vi "Start Continuous Acquisition.vi"(6 "lpszRefPath":string, 7 "nMode":u32, 8 "error in (no error)":errorcluster, 9 "pImg":u16[](array[numeric]), 10 "refImg":u16[](array[numeric]), 11 "nSensorIP":u32) -> (0 "error out":errorcluster, 1 "pImg out":u16[](array[numeric]), 2 "refImg out":u16[](array[numeric]), 3 "function return":i32)   [LabVIEW 2017, in "BonTechWrapperLibrary.lvlib"]
doc: "extern \"C\" BONTECHLIBRARY_API int __stdcall StartContinuousAcquisition(unsigned int nSensorIP);\nextern \"C\" BONTECHLIBRARY_API int __stdcall StartContinuousAcquisition(unsigned int nSensorIP, unsigned short* pImg, unsigned int nMode, LPCTSTR lpszRefPath);\n\nextern \"C\" BONTECHLIBRARY_API int __stdcall StartContinuousAcquisition(unsigned int nSensorIP, unsigned short* refImg, unsigned short* pImg, unsigned int nMode, LPCTSTR lpszRefPath);"
uses:
  BonTechWrapperLibrary.lvlib
  BonTechWrapperLibrary.dll
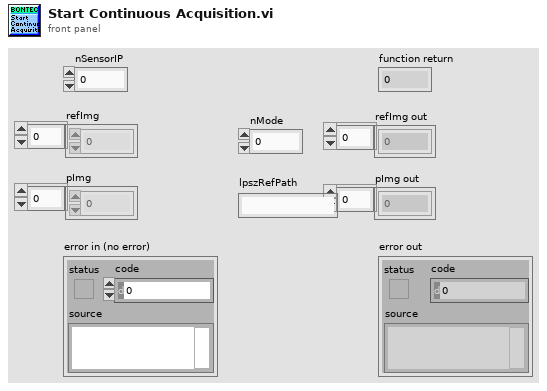
[diagram p1: front panel]
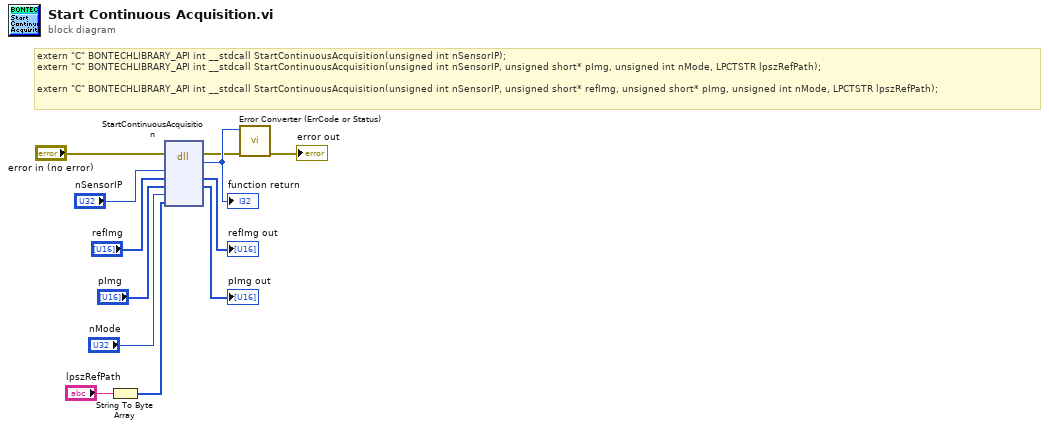
[diagram p0: block diagram]
diagram:
  # "extern \"C\" BONTECHLIBRARY_API int __stdcall StartContinuousAcquisition(unsigned int nSensorIP);\nextern \"C\" BONTECHLIBRARY_API int __stdcall StartContinuousAcquisition(unsigned int nSensorIP, unsigned short* pImg, unsigned int nMode, LPCTSTR lpszRefPath);\n\nextern \"C\" BONTECHLIBRARY_API int __stdcall StartContinuousAcquisition(unsigned int nSensorIP, unsigned short* refImg, unsigned short* pImg, unsigned int nMode, LPCTSTR lpszRefPath);"
  n1 = String To Byte Array(string="lpszRefPath") -> (unsigned byte array=w1:u8[])
  n2 = dll-call lib="C:/Users/Achuthaperumal/SourceCodes/BonTechWrapperLibrary/BonTechWrapperLibrary/x64/Release/BonTechWrapperLibrary.*" fn="StartContinuousAcquisition"(error in="error in (no error)", "nSensorIP"="nSensorIP", "refImg"="refImg", "pImg"="pImg", "nMode"="nMode", "lpszRefPath"=w1) -> (error out=w3:errorcluster, "return type"=w12:i32, "refImg"=→"refImg out":u16[], "pImg"=→"pImg out":u16[])  [unwired: 5 in, 1 out]
  "function return" <- w12
  n3 = call "Error Converter (ErrCode or Status).vi"("error in (no error)"=w3, "error code"=w12) -> ("error out"=→"error out":errorcluster)  [unwired: 9 in]
